vi "Data Latch Master.vi"(4 "Need to Receive In":bool, 5 "Need to Send In":bool, 6 "FPGA's Data Latch":T1, 7 "RT's Data Latch In":T1) -> (0 "Need to Receive Out":bool, 1 "Need to Send Out":bool, 2 "Done":bool, 3 "RT's Data Latch Out":T1)   [LabVIEW 2010]
uses:
  2-Low Neurons/Data Latch.ctl
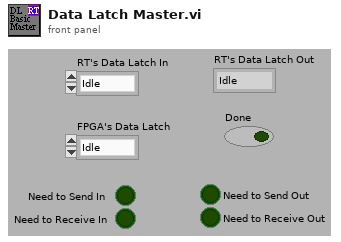
[diagram p1: front panel]
types:
  T1 = typedef "Data Latch.ctl" = enum8{"Idle", "Sending", "Sent", "Receiving", "Received"}
  T2 = enum8{"Idle", "Sending", "Sent", "Receiving", "Received"}
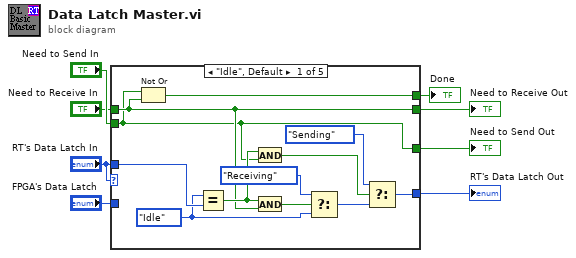
[diagram p0: block diagram]
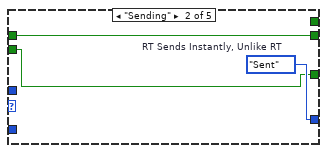
[diagram p2: hidden frame]
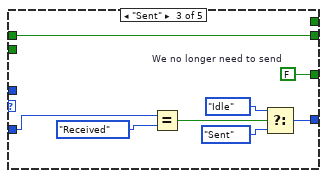
[diagram p3: hidden frame]
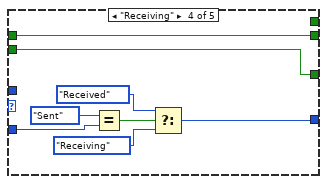
[diagram p4: hidden frame]
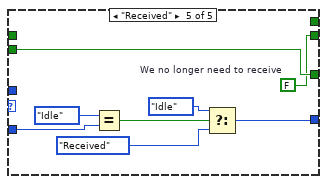
[diagram p5: hidden frame]
diagram:
  n1 = case shown="\"Idle\", Default" "RT's Data Latch In" {
    tunnel: "FPGA's Data Latch" -> [_ _ w31 w36 w47]
    tunnel: [w13 w23 w29 w37 w45] -> w8
    tunnel: "Need to Send In" -> [w10 w22 _ w32 w41]
    tunnel: "Need to Receive In" -> [w11 w21 w26 w33 _]
    tunnel: "RT's Data Latch In" -> [w18 _ _ _ _]
    tunnel: [w10 w22 w27 w32 w41] -> w3
    tunnel: [w11 w21 w26 w33 w40] -> w2
    tunnel: [w9 _ _ _ _] -> w1
    frame "Idle", Default {
      w12 = Data_Latch."Idle" ("Data Latch")
      n2 = Not Or(1:w11, 2:w10) -> (0:w9:bool)
      n3 = Equal?(x=w12, y=w18) -> (x = y?=w16:bool)
      n4 = And(x=w16, y=w10) -> (x .and. y?=w20:bool)
      n5 = And(x=w16, y=w11) -> (x .and. y?=w15:bool)
      n6 = Select(t=Data_Latch."Receiving", s=w15, f=w12) -> (s? t:f=w14:T1)
      n7 = Select(t=Data_Latch."Sending", s=w20, f=w14) -> (s? t:f=w13:T1)
    }
    frame "Sending" {
      w23 = Data_Latch."Sent"  # RT Sends Instantly, Unlike RT
    }
    frame "Sent" {
      w27 = FALSE  # We no longer need to send
      n8 = Equal?(x=w31, y=T2."Received") -> (x = y?=w28:bool)
      n9 = Select(t=Data_Latch."Idle", s=w28, f=Data_Latch."Sent") -> (s? t:f=w29:T1)
    }
    frame "Receiving" {
      n10 = Equal?(x=T2."Sent", y=w36) -> (x = y?=w38:bool)
      n11 = Select(t=Data_Latch."Received", s=w38, f=Data_Latch."Receiving" ("RT's Data Latch In")) -> (s? t:f=w37:T1)
    }
    frame "Received" {
      w40 = FALSE  # We no longer need to receive
      n12 = Equal?(x=T2."Idle", y=w47) -> (x = y?=w44:bool)
      n13 = Select(t=Data_Latch."Idle", s=w44, f=Data_Latch."Received") -> (s? t:f=w45:T1)
    }
  }
  "Done" <- w1
  "RT's Data Latch Out" <- w8
  "Need to Send Out" <- w3
  "Need to Receive Out" <- w2
